vi "Teleop.vi"(10 "Match Info":T1={"Autonomous Elapsed Seconds"=0.0, "TeleOp Elapsed Seconds"=0.0, "Disabled Elapsed Seconds"=0.0, "Visited Autonomous"=FALSE, "Visited TeleOp"=FALSE, "Visited Disabled"=FALSE, "Autonomous Settings"={"Autonomous Style"=enum."Independent", "VI Refnum"=refnum}}, 11 "Call Context":T2=enum."Stop") -> ()   [LabVIEW 2015]
doc: "This VI is called for each TeleOp packet received from the DS where the robot is not disabled. It is often used to read from the joysticks and update I/O or to update setpoints for timed control loops. It should complete and return within 20 milliseconds or it may miss DS packets."
uses:
  <vilib>/Rock Robotics/WPI/DriverStation/WPI_DriverStationDerivedRobotMode.ctl
  <vilib>/Rock Robotics/WPI/DriverStation/WPI_DriverStationMatch Info.ctl
  Typedef/XBox Buttons.ctl
  Typedef/XBox Axis.ctl
  <vilib>/Rock Robotics/WPI/Utilities/WPI_GetSetVariantRefNum.vi
  <vilib>/Rock Robotics/Network Tables/NT Write Boolean Array.vi
  <vilib>/Rock Robotics/Network Tables/NT Write Numeric Array.vi
  Robot Global Data.vi
  <vilib>/Rock Robotics/WPI/RobotDrive/WPI_RobotDriveArcadeDrive_Standard(NoSaturation).vi
  <vilib>/Rock Robotics/Network Tables/NT Write Number.vi
  ArmController/ArmController.lvlib
  <vilib>/Rock Robotics/WPI/Solenoid/WPI_SolenoidSetEnum.vi
  <vilib>/Rock Robotics/WPI/Solenoid/WPI_SolenoidValue.ctl
panel:
  in  "Position":dbl caption="Test Servo Position"
  in  "ServoClose":dbl
  in  "Servo Open":dbl
  in  "Allow Hang":bool
  in  "Winch Speed":dbl=1.0 format="%#_13g"
  in  "Match Time":dbl=115.0 format="%#_13g"
  in  "Reset":bool
  out "Shifts":i32
  # "Hanger"
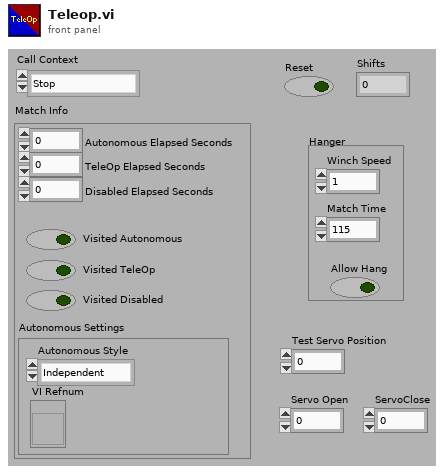
[diagram p1: front panel]
types:
  T1 = typedef "WPI_DriverStationMatch Info.ctl" = cluster{"Autonomous Elapsed Seconds":dbl, "TeleOp Elapsed Seconds":dbl, "Disabled Elapsed Seconds":dbl, "Visited Autonomous":bool, "Visited TeleOp":bool, "Visited Disabled":bool, "Autonomous Settings":cluster{"Autonomous Style":enum16{"Iterative", "Independent"}, "VI Refnum":refnum<vi>}}
  T2 = typedef "WPI_DriverStationDerivedRobotMode.ctl" = enum16{"Init", "Execute", "Stop"}
  T3 = typedef "XBox Buttons.ctl" = enum16{"A", "B", "X", "Y", "Left Bumper", "Right Bumper", "Back", "Start", "Left Joystick", "Right Joystick"}
  T4 = typedef "XBox Axis.ctl" = enum16{"Left X", "Left Y", "Left Trigger", "Right Trigger", "Right X", "Right Y"}
  T5 = typedef "WPI_RobotDriveDevRef.ctl" = cluster{"DevStatus":errorcluster, "Motors[]":T6[], "Square Inputs":bool, "Max Output":dbl}
  T6 = typedef "WPI_MotorControlDeviceRef.ctl" = cluster{"DeviceStatus":errorcluster, "Type":T7, "PWM":cluster{"PWM Channel":T8, "DeadBand":T9}, "CAN":cluster{"Device Number":u8, "Control Mode":T10, "Semaphore":T11, "Max Vout":dbl, "TalonSRX Control Mode":T12}, "Invert":bool}
  T7 = typedef "WPI_MotorControlType.ctl" = enum16{"PWM", "CAN", "CANTalonSRX"}
  T8 = typedef "FPGA_DIOPWMChannel.ctl" = enum8{"PWM 0", "PWM 1", "PWM 2", "PWM 3", "PWM 4", "PWM 5", "PWM 6", "PWM 7", "PWM 8", "PWM 9", "PWM MXP 0", "PWM MXP 1", "PWM MXP 2", "PWM MXP 3", "PWM MXP 4", "PWM MXP 5", "PWM MXP 6", "PWM MXP 7", "PWM MXP 8", "PWM MXP 9", "Invalid"}
  T9 = typedef "WPI_PWMDeadband.ctl" = cluster{"Name":string, "maxPositivePwm":i32, "minPositivePwm":i32, "centerPwm":i32, "maxNegativePwm":i32, "minNegativePwm":i32, "angularRange":u16}
  T10 = typedef "WPI_CANJaguar_ControlMode.ctl" = enum8{"Percent VBus", "Current", "Speed", "Position", "Voltage"}
  T11 = typedef "Semaphore RefNum" = refnum<k1>
  T12 = typedef "WPI_CANTalonSRX_APIControlMode.ctl" = enum8{"Percent VBus", "Speed", "Position", "Slave", "Unchanged / Invalid", "Voltage Compensation", "Current", "Motion Profile"}
  T13 = typedef "WPI_JoystickDevRef.ctl" = cluster{"Device":T14}
  T14 = typedef "WPI_JoystickDeviceEnum.ctl" = enum16{"USB 0", "USB 1", "USB 2", "USB 3", "USB 4", "USB 5"}
  T15 = typedef "WPI_SolenoidValue.ctl" = enum16{"Off", "On", "Forward", "Reverse"}
  T16 = typedef "ArmController.lvlib/ArmRef.ctl" = cluster{"Pot":T17, "ArmMotor":T6, "Queue":refnum<queue>, "Setpoint":dbl, "Manual":bool, "output range":cluster{"output high":dbl, "output low":dbl}, "PID gains":cluster{"proportional gain (Kc)":dbl, "integral time (Ti, min)":dbl, "derivative time (Td, min)":dbl}}
  T17 = typedef "WPI_PotentiometerDevRef.ctl" = cluster{"DevStatus":errorcluster, "Analog Channel":T18, "Invert Output":bool}
  T18 = typedef "FPGA_AIChannel.ctl" = enum8{"AI 0", "AI 1", "AI 2", "AI 3", "AI MXP 0", "AI MXP 1", "AI MXP 2", "AI MXP 3", "Invalid"}
  T19 = typedef "WPI_ServoDeviceRef.ctl" = cluster{"DeviceStatus":errorcluster, "PWM Channel":T8, "DeadBand":T9}
  T20 = cluster{"Down":dbl, "Pickup":dbl, "Shoot":dbl, "Turtle":dbl, "Intake Block":dbl, "Intake Transfer":dbl, "Cheval De Fris":dbl, "Hang":dbl}
  T21 = cluster{"Down":dbl, "Pickup":dbl, "Shoot":dbl, "Turtle":dbl, "Intake Transfer":dbl, "Hang":dbl}
  T22 = typedef "WPI_SolenoidDevRef.ctl" = cluster{"DevStatus":errorcluster, "Pneumatics Control Module":u8, "Forward Solenoid Channel":T23, "Reverse Solenoid Channel":T23}
  T23 = typedef "WPI_SolenoidChannel.ctl" = enum8{"Solenoid 0", "Solenoid 1", "Solenoid 2", "Solenoid 3", "Solenoid 4", "Solenoid 5", "Solenoid 6", "Solenoid 7", "Invalid"}
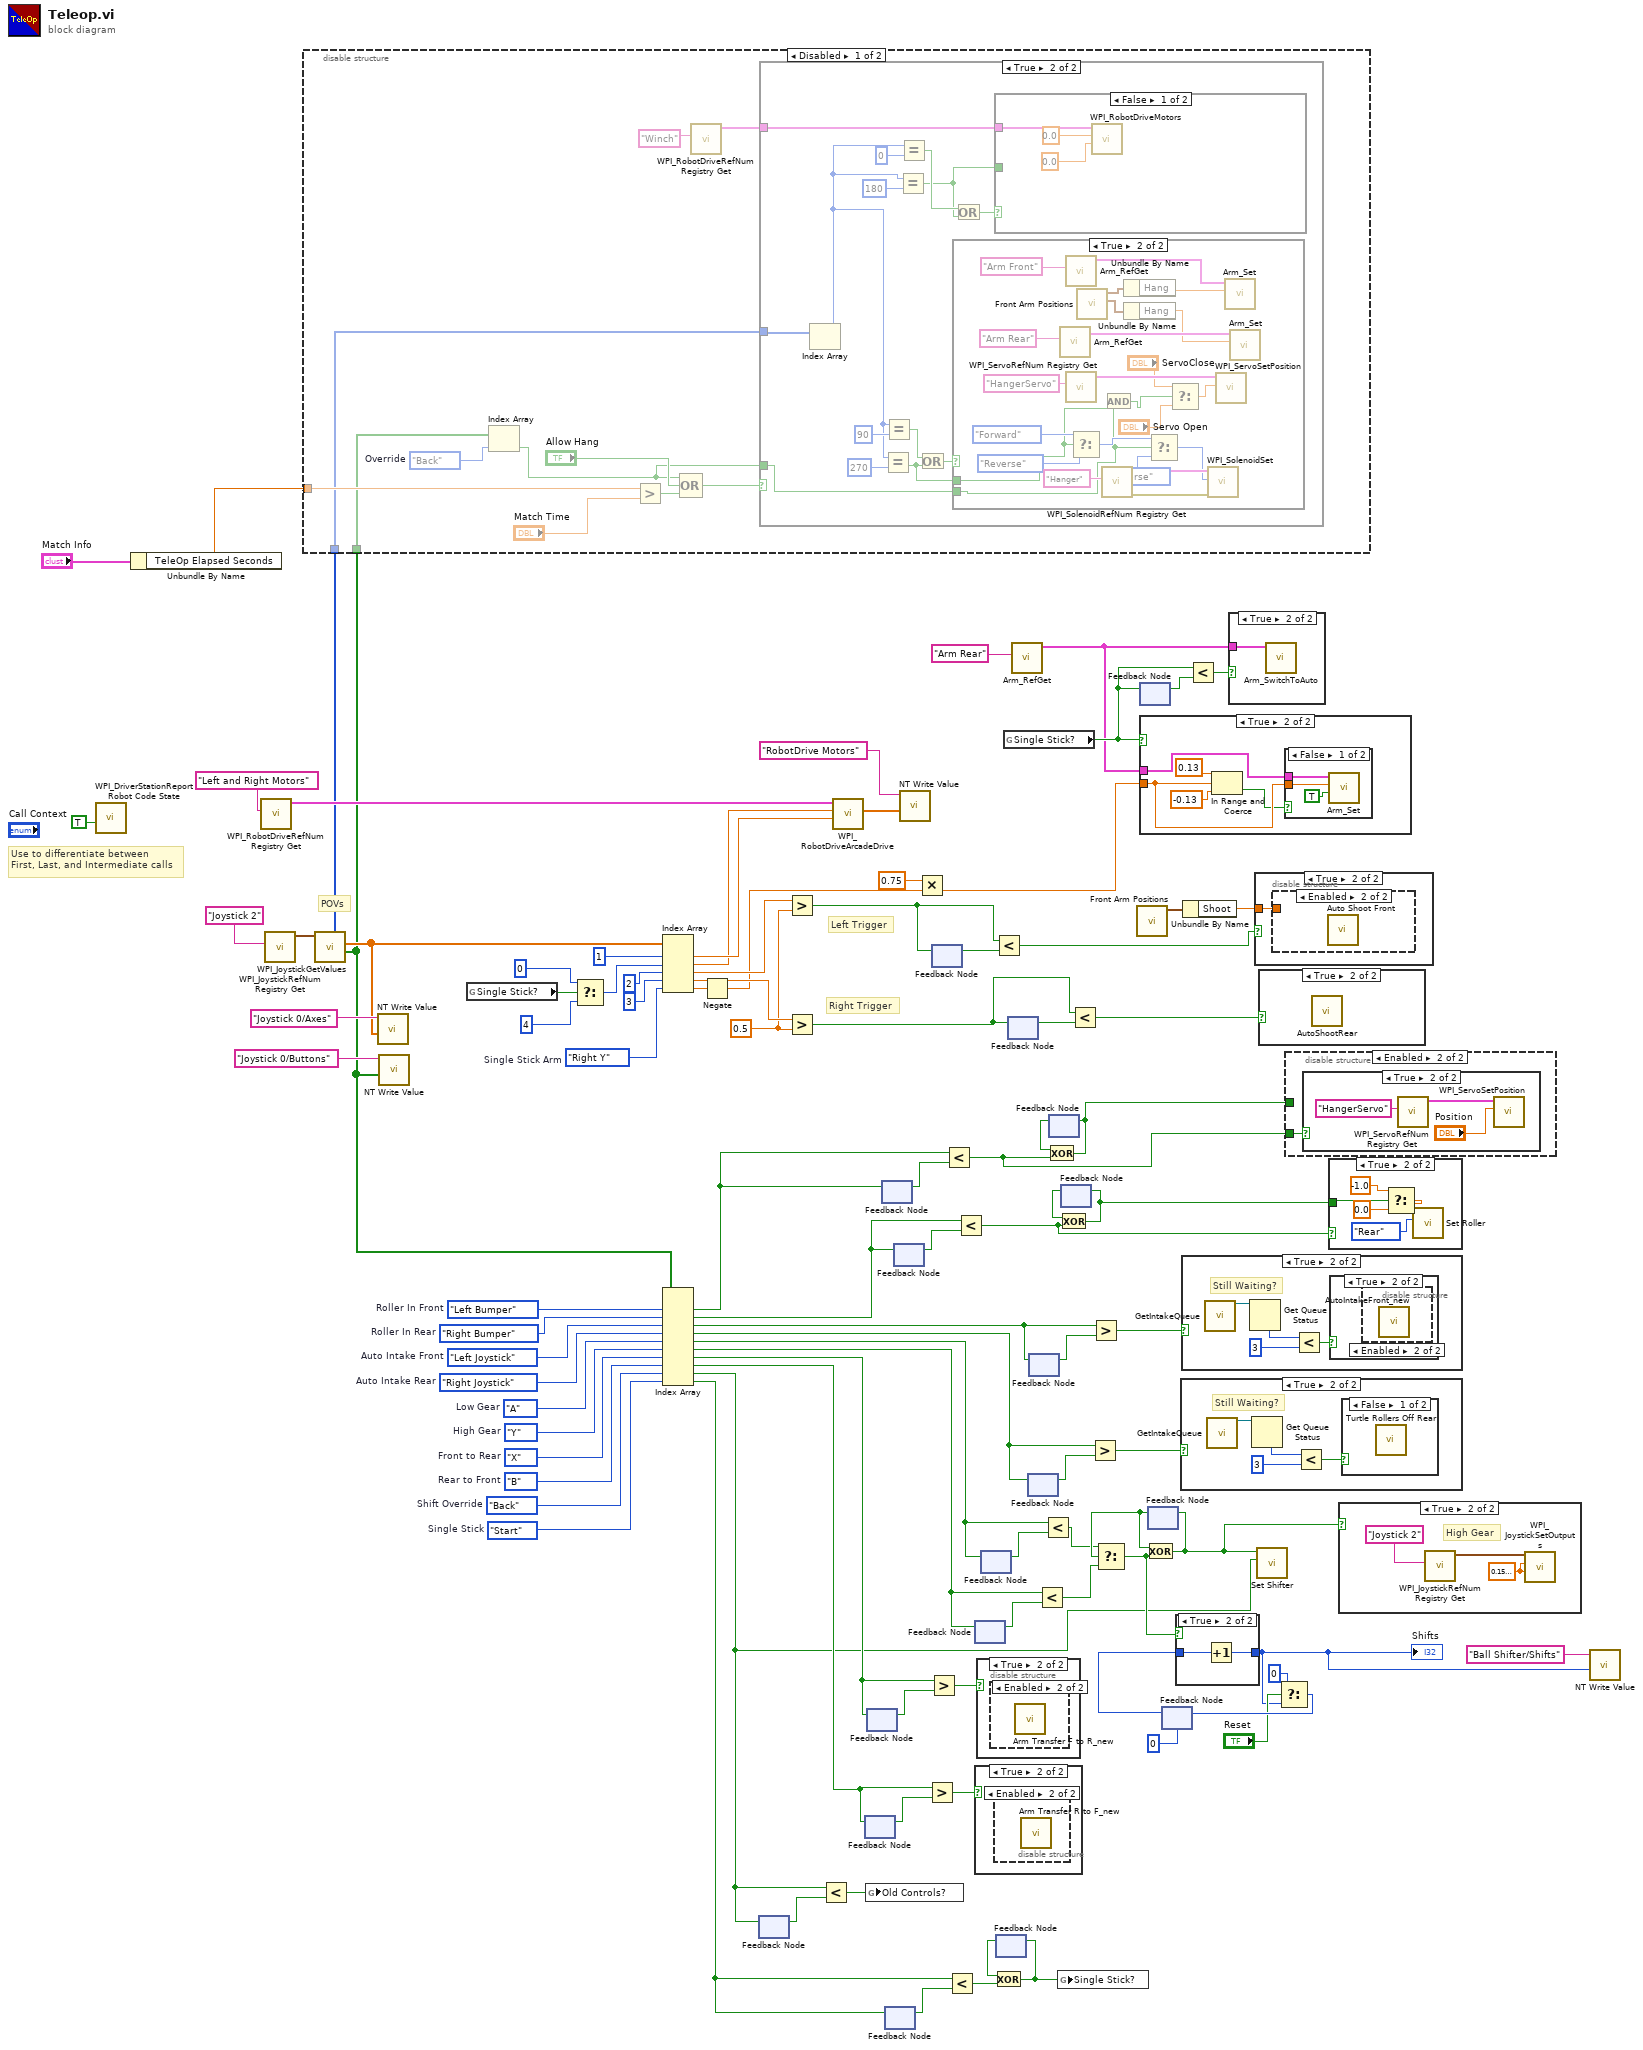
[diagram p0: block diagram]
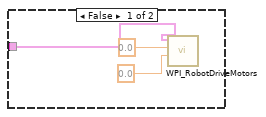
[diagram p2: hidden frame]
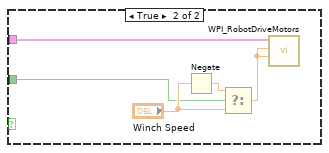
[diagram p4: hidden frame]
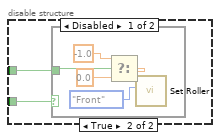
[diagram p6: hidden frame]
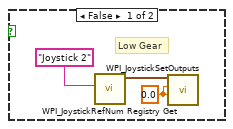
[diagram p9: hidden frame]
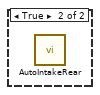
[diagram p11: hidden frame]
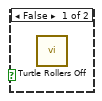
[diagram p13: hidden frame]
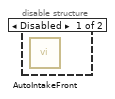
[diagram p14: hidden frame]
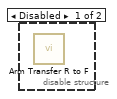
[diagram p16: hidden frame]
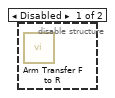
[diagram p20: hidden frame]
diagram:
  w44 = XBox_Buttons."Left Bumper"  # Roller In Front
  w43 = XBox_Buttons."Right Bumper"  # Roller In Rear
  w50 = XBox_Axis."Right Y"  # Single Stick Arm
  w51 = XBox_Buttons."Left Joystick"  # Auto Intake Front
  w52 = XBox_Buttons."Right Joystick"  # Auto Intake Rear
  w53 = XBox_Buttons."A"  # Low Gear
  w54 = XBox_Buttons."Y"  # High Gear
  w55 = XBox_Buttons."X"  # Front to Rear
  w56 = XBox_Buttons."B"  # Rear to Front
  w57 = XBox_Buttons."Back"  # Shift Override
  w58 = XBox_Buttons."Start"  # Single Stick
  w79 = 0.5 ("x")
  # "POVs"
  # "Right Trigger"
  # "Left Trigger"
  # "Use to differentiate between\nFirst, Last, and Intermediate calls"
  n1 = call <vilib>:"WPI_DriverStationReport Robot Code State.vi"("TeleOp"=TRUE ("Autonomous")) -> ()  [unwired: 10 in, 1 out]
  n2 = Unbundle By Name("Match Info") -> ("TeleOp Elapsed Seconds"=w3:dbl)
  n3 = call <vilib>:"WPI_RobotDriveRefNum Registry Get.vi"("refnum name"="Left and Right Motors") -> ("RobotDriveDevRef"=w99:T5)  [unwired: 1 in, 9 out]
  n4 = call <vilib>:"WPI_JoystickRefNum Registry Get.vi"("refnum name"="Joystick 2") -> ("JoystickDevRef"=w6:T13)  [unwired: 1 in, 9 out]
  n5 = call <vilib>:"WPI_JoystickGetValues.vi"("JoystickDevRef"=w6) -> ("Buttons"=w2:bool[], "Axes"=w82:dbl[], "POVs"=w1:i16[])  [unwired: 6 in, 2 out]
  n6 = disable-structure shown="Disabled" {
    disable-tunnel: w3 -> [w111 _]
    disable-tunnel: w2 -> [w105 _]
    disable-tunnel: w1 -> [w104 _]
    frame Disabled {
      w106 = XBox_Buttons."Back"  # Override
      n7 = Index Array(array=w105, index=w106) -> (element=w103:bool)
      n8 = Greater?(x=w111, y="Match Time") -> (0:w108:bool)
      n9 = Compound Arithmetic op=OR(w103, "Allow Hang", w108) -> (w109:bool)
      n10 = call <vilib>:"WPI_RobotDriveRefNum Registry Get.vi"("refnum name"="Winch") -> ("RobotDriveDevRef"=w101:T5)  [unwired: 1 in, 9 out]
      n11 = case shown="True" w109 {
        tunnel: w104 -> [_ w126]
        tunnel: w103 -> [_ w116]
        tunnel: w101 -> [w112 w115]
        frame False {
          n12 = call <vilib>:"WPI_RobotDriveMotors.vi"("RightSpeed"=0.0, "LeftSpeed"=0.0, "RobotDriveDevRef"=w112) -> ()  [unwired: 6 in, 3 out]
        }
        frame True {
          n13 = Index Array(array=w126) -> (element=w121:i16)  [unwired: 1 in]
          n14 = Equal?(x=w121, y=i16 270) -> (x = y?=w117:bool)
          n15 = Equal?(x=w121, y=i16 90) -> (x = y?=w120:bool)
          n16 = Equal?(x=w121, y=i16 180) -> (x = y?=w118:bool)
          n17 = Equal?(x=w121, y=i16 0) -> (x = y?=w119:bool)
          n18 = Or(x=w120, y=w117) -> (x .or. y?=w127:bool)
          n19 = case shown="True" w127 {
            tunnel: w117 -> [_ w132]
            tunnel: w116 -> [_ w133]
            frame False {
            }
            frame True {
              n20 = call "Arm_RefGet.vi"("refnum name"="Arm Rear") -> ("ArmRef"=w144:T16)  [unwired: 9 in, 1 out]
              n21 = call "Arm_RefGet.vi"("refnum name"="Arm Front") -> ("ArmRef"=w145:T16)  [unwired: 9 in, 1 out]
              n22 = call <vilib>:"WPI_ServoRefNum Registry Get.vi"("refnum name"="HangerServo") -> ("ServoDeviceRef"=w135:T19)  [unwired: 9 in, 1 out]
              n23 = Select(t=WPI_SolenoidValue."Forward" ("Direction"), s=w132, f=WPI_SolenoidValue."Reverse" ("Direction")) -> (s? t:f=w139:T15)
              n24 = call "Front Arm Positions.vi"() -> ("Rear Arm"=w148:T20, "Front Arm"=w149:T21)  [unwired: 10 in]
              n25 = call <vilib>:"WPI_SolenoidRefNum Registry Get.vi"("refnum name"="Hanger") -> ("error out"=w150:errorcluster, "SolenoidDevRef"=w152:T22)  [unwired: 9 in]
              n26 = And(x=w132, y=w133) -> (x .and. y?=w134:bool)
              n27 = Unbundle By Name(w149) -> ("Hang"=w142:dbl)
              n28 = Unbundle By Name(w148) -> ("Hang"=w143:dbl)
              n29 = Select(t=w139, s=w133, f=WPI_SolenoidValue."Reverse" ("Direction")) -> (s? t:f=w137:T15)
              n30 = Select(t="ServoClose", s=w134, f="Servo Open") -> (s? t:f=w131:dbl)
              n31 = call-poly <vilib>:"WPI_SolenoidSet.vi"("error in (no error)"=w150, "Value"=w137, "SolenoidDevRef"=w152) -> ()  [unwired: 7 in, 2 out]
              n32 = call <vilib>:"WPI_ServoSetPosition.vi"("Position"=w131, "ServoDeviceRef"=w135) -> ()  [unwired: 8 in, 2 out]
              n33 = call "Arm_Set.vi"("Value"=w142, "ArmRef in"=w145) -> ()  [unwired: 8 in, 2 out]
              n34 = call "Arm_Set.vi"("Value"=w143, "ArmRef in"=w144) -> ()  [unwired: 8 in, 2 out]
            }
          }
          n35 = Or(x=w119, y=w118) -> (x .or. y?=w128:bool)
          n36 = case shown="False" w128 {
            tunnel: w118 -> [_ w157]
            tunnel: w115 -> [w155 w156]
            frame False {
              n37 = call <vilib>:"WPI_RobotDriveMotors.vi"("RightSpeed"=0.0, "LeftSpeed"=0.0, "RobotDriveDevRef"=w155) -> ()  [unwired: 6 in, 3 out]
            }
            frame True {
              n38 = Negate(x="Winch Speed") -> (-x=w159:dbl)
              n39 = Select(t=w159, s=w157, f="Winch Speed") -> (s? t:f=w160:dbl)
              n40 = call <vilib>:"WPI_RobotDriveMotors.vi"("RightSpeed"=w160, "LeftSpeed"=w160, "RobotDriveDevRef"=w156) -> ()  [unwired: 6 in, 3 out]
            }
          }
        }
      }
    }
    frame Enabled {
    }
  }
  n41 = call-poly <vilib>:"NT Write Value.vi"("Numeric Array"=w82, "Name"="Joystick 0/Axes") -> ()  [unwired: 9 in, 1 out]
  n42 = call-poly <vilib>:"NT Write Value.vi"("Boolean Array"=w2, "Name"="Joystick 0/Buttons") -> ()  [unwired: 9 in, 1 out]
  n43 = global read "Robot Global Data.vi" "Single Stick?"() -> (w62:bool)
  n44 = Select(t=0 ("index"), s=w62, f=4 ("index")) -> (s? t:f=w59:i32)
  n45 = Index Array(array=w82, index #1=1 ("index"), index #2=w59, index #3=2 ("index"), index #4=3 ("index"), index #5=w50) -> (element #1=w97:dbl, element #2=w94:dbl, element #3=w81:dbl, element #4=w80:dbl, element #5=w66:dbl)
  n46 = Index Array(array=w2, index #1=w44, index #2=w43, index #3=w51, index #4=w52, index #5=w53, index #6=w54, index #7=w55, index #8=w56, index #9=w57, index #10=w58) -> (element #1=w29:bool, element #2=w28:bool, element #3=w48:bool, element #4=w45:bool, element #5=w41:bool, element #6=w37:bool, element #7=w20:bool, element #8=w9:bool, element #9=w5:bool, element #10=w73:bool)
  n47 = Negate(x=w66) -> (-x=w12:dbl)
  n48 = feedback #1() -> (w35:bool)  [unwired: 1 in]
  n49 = feedback-in #1(w5) -> ()
  n50 = Greater?(x=w81, y=w79) -> (0:w24:bool)
  n51 = Greater?(x=w80, y=w79) -> (0:w17:bool)
  n52 = Less?(x=w5, y=w35) -> (x < y?=w34:bool)
  n53 = call-poly <vilib>:"WPI_RobotDriveArcadeDrive.vi"("Y axis value"=w97, "X axis value"=w94, "RobotDriveDevRef"=w99) -> ("Motor Values"=w96:dbl[])  [unwired: 6 in, 2 out]
  n54 = feedback #2() -> (w10:bool)  [unwired: 1 in]
  n55 = feedback-in #2(w9) -> ()
  n56 = global write "Robot Global Data.vi" "Old Controls?"(w34) -> ()
  n57 = feedback #3() -> (w22:bool)  [unwired: 1 in]
  n58 = feedback-in #3(w20) -> ()
  n59 = feedback #4() -> (w33:bool)  [unwired: 1 in]
  n60 = feedback-in #4(w29) -> ()
  n61 = feedback #5() -> (w74:bool)  [unwired: 1 in]
  n62 = feedback-in #5(w73) -> ()
  n63 = feedback #6() -> (w30:bool)  [unwired: 1 in]
  n64 = feedback-in #6(w28) -> ()
  n65 = call-poly <vilib>:"NT Write Value.vi"("Numeric Array"=w96, "Name"="RobotDrive Motors") -> ()  [unwired: 9 in, 1 out]
  n66 = Multiply(x=0.75, y=w12) -> (x*y=w8:dbl)
  n67 = Greater?(x=w9, y=w10) -> (0:w11:bool)
  n68 = Greater?(x=w20, y=w22) -> (0:w21:bool)
  n69 = feedback #7() -> (w25:bool)  [unwired: 1 in]
  n70 = feedback-in #7(w24) -> ()
  n71 = Less?(x=w29, y=w33) -> (x < y?=w16:bool)
  n72 = Less?(x=w73, y=w74) -> (x < y?=w76:bool)
  n73 = Less?(x=w28, y=w30) -> (x < y?=w13:bool)
  n74 = feedback #8() -> (w39:bool)  [unwired: 1 in]
  n75 = feedback-in #8(w37) -> ()
  n76 = case shown="True" w11 {
    frame False {
    }
    frame True {
      n77 = disable-structure shown="Enabled" {
        frame Disabled {
          n78 = call "Arm Transfer R to F.vi"() -> ()  [unwired: 12 in]
        }
        frame Enabled {
          n79 = call "Arm Transfer R to F_new.vi"() -> ()  [unwired: 12 in]
        }
      }
    }
  }
  n80 = case shown="True" w21 {
    frame False {
    }
    frame True {
      n81 = disable-structure shown="Enabled" {
        frame Disabled {
          n82 = call "Arm Transfer F to R.vi"() -> ()  [unwired: 12 in]
        }
        frame Enabled {
          n83 = call "Arm Transfer F to R_new.vi"() -> ()  [unwired: 12 in]
        }
      }
    }
  }
  n84 = feedback #9() -> (w93:bool)  [unwired: 1 in]
  n85 = feedback-in #9(w41) -> ()
  n86 = Less?(x=w24, y=w25) -> (x < y?=w23:bool)
  n87 = feedback #10() -> (w75:bool)  [unwired: 1 in]
  n88 = Exclusive Or(1:w76, 2:w75) -> (0:w72:bool)
  n89 = feedback-in #10(w72) -> ()
  n90 = global read "Robot Global Data.vi" "Single Stick?"() -> (w70:bool)
  n91 = feedback #11() -> (w19:bool)  [unwired: 1 in]
  n92 = feedback-in #11(w17) -> ()
  n93 = call "Arm_RefGet.vi"("refnum name"="Arm Rear") -> ("ArmRef"=w67:T16)  [unwired: 9 in, 1 out]
  n94 = feedback #12() -> (w46:bool)  [unwired: 1 in]
  n95 = feedback-in #12(w45) -> ()
  n96 = feedback #13() -> (w87:bool)  [unwired: 1 in]
  n97 = feedback-in #13(w48) -> ()
  n98 = Less?(x=w37, y=w39) -> (x < y?=w38:bool)
  n99 = Less?(x=w41, y=w93) -> (x < y?=w40:bool)
  n100 = feedback #14() -> (w32:bool)  [unwired: 1 in]
  n101 = Exclusive Or(1:w16, 2:w32) -> (0:w15:bool)
  n102 = feedback-in #14(w15) -> ()
  n103 = global write "Robot Global Data.vi" "Single Stick?"(w72) -> ()
  n104 = feedback #15() -> (w31:bool)  [unwired: 1 in]
  n105 = Exclusive Or(1:w13, 2:w31) -> (0:w14:bool)
  n106 = feedback-in #15(w14) -> ()
  n107 = Less?(x=w17, y=w19) -> (x < y?=w18:bool)
  n108 = Greater?(x=w45, y=w46) -> (0:w47:bool)
  n109 = Greater?(x=w48, y=w87) -> (0:w49:bool)
  n110 = call "Front Arm Positions.vi"() -> ("Front Arm"=w27:T21)  [unwired: 10 in, 1 out]
  n111 = feedback #16() -> (w71:bool)  [unwired: 1 in]
  n112 = feedback-in #16(w70) -> ()
  n113 = case shown="True" w70 {
    tunnel: w67 -> [_ w163]
    tunnel: w8 -> [_ w162]
    frame False {
    }
    frame True {
      n114 = In Range and Coerce(upper limit=0.13, x=w162, lower limit=-0.13) -> (In Range?=w161:bool)  [unwired: 1 out]
      n115 = case shown="False" w161 {
        tunnel: w163 -> [w168 w169]
        tunnel: w162 -> [w167 _]
        frame False {
          n116 = call "Arm_Set.vi"("Manual Control"=TRUE, "Value"=w167, "ArmRef in"=w168) -> ()  [unwired: 7 in, 2 out]
        }
        frame True {
          n117 = call "Arm_SwitchToAuto.vi"("ArmRef in"=w169) -> ()  [unwired: 9 in, 2 out]
        }
      }
    }
  }
  n118 = feedback #17() -> (w42:bool)  [unwired: 1 in]
  n119 = Select(t=w40, s=w42, f=w38) -> (s? t:f=w36:bool)
  n120 = Exclusive Or(1:w36, 2:w42) -> (0:w4:bool)
  n121 = feedback-in #17(w4) -> ()
  n122 = feedback #18(0) -> (w91:i32)
  n123 = case shown="True" w36 {
    tunnel: w91 -> [w170 w172]
    tunnel: [w170 w171] -> w78
    frame False {
    }
    frame True {
      n124 = Increment(x=w172) -> (x+1=w171:i32)
    }
  }
  "Shifts" <- w78
  n125 = case shown="True" w47 {
    frame False {
    }
    frame True {
      # "Still Waiting?"
      n126 = call "GetIntakeQueue.vi"() -> ("queue out"=w174:refnum<queue>)  [unwired: 11 in]
      n127 = Get Queue Status(queue=w174) -> (# elements in queue=w175:i32)  [unwired: 2 in, 7 out]
      n128 = Less?(x=w175, y=3) -> (x < y?=w173:bool)
      n129 = case shown="False" w173 {
        frame False {
          n130 = call "Turtle Rollers Off Rear.vi"() -> ()  [unwired: 12 in]
        }
        frame True {
          n131 = call "AutoIntakeRear.vi"() -> ()  [unwired: 12 in]
        }
      }
    }
  }
  n132 = case shown="True" w49 {
    frame False {
    }
    frame True {
      # "Still Waiting?"
      n133 = call "GetIntakeQueue.vi"() -> ("queue out"=w180:refnum<queue>)  [unwired: 11 in]
      n134 = Get Queue Status(queue=w180) -> (# elements in queue=w179:i32)  [unwired: 2 in, 7 out]
      n135 = Less?(x=w179, y=3) -> (x < y?=w177:bool)
      n136 = case shown="True" w177 {
        frame False {
          n137 = call "Turtle Rollers Off.vi"() -> ()  [unwired: 12 in]
        }
        frame True {
          n138 = disable-structure shown="Enabled" {
            frame Disabled {
              n139 = call "AutoIntakeFront.vi"() -> ()  [unwired: 12 in]
            }
            frame Enabled {
              n140 = call "AutoIntakeFront_new.vi"() -> ()  [unwired: 12 in]
            }
          }
        }
      }
    }
  }
  n141 = Unbundle By Name(w27) -> ("Shoot"=w26:dbl)
  n142 = Less?(x=w70, y=w71) -> (x < y?=w69:bool)
  n143 = case shown="True" w69 {
    tunnel: w67 -> [_ w181]
    frame False {
    }
    frame True {
      n144 = call "Arm_SwitchToAuto.vi"("ArmRef in"=w181) -> ()  [unwired: 9 in, 2 out]
    }
  }
  n145 = case shown="True" w23 {
    tunnel: w26 -> [_ w182]
    frame False {
    }
    frame True {
      n146 = disable-structure shown="Enabled" {
        disable-tunnel: w182 -> [w184 _]
        frame Disabled {
          n147 = call "Set Arm.vi"("Intake"=enum16{"Front", "Rear"}."Front", "Position"=w184) -> ()  [unwired: 10 in]
        }
        frame Enabled {
          n148 = call "Auto Shoot Front.vi"() -> ()  [unwired: 12 in]
        }
      }
    }
  }
  n149 = call "Set Shifter.vi"("Override?"=w5, "Gear (F = Low Gear)"=w4) -> ()  [unwired: 9 in, 1 out]
  n150 = case shown="True" w18 {
    frame False {
    }
    frame True {
      n151 = call "AutoShootRear.vi"() -> ()  [unwired: 12 in]
    }
  }
  n152 = Select(t=0, s="Reset", f=w78) -> (s? t:f=w89:i32)
  n153 = feedback-in #18(w89) -> ()
  n154 = disable-structure shown="Enabled" {
    disable-tunnel: w16 -> [w186 w192]
    disable-tunnel: w15 -> [w185 _]
    frame Disabled {
      n155 = case shown="True" w186 {
        tunnel: w185 -> [_ w190]
        frame False {
        }
        frame True {
          n156 = Select(t=-1.0 ("Speed"), s=w190, f=0.0) -> (s? t:f=w188:dbl)
          n157 = call "Set Roller.vi"("Intake"=enum16{"Front", "Rear"}."Front", "Speed"=w188) -> ()  [unwired: 10 in]
        }
      }
    }
    frame Enabled {
      n158 = case shown="True" w192 {
        frame False {
        }
        frame True {
          n159 = call <vilib>:"WPI_ServoRefNum Registry Get.vi"("refnum name"="HangerServo") -> ("ServoDeviceRef"=w194:T19)  [unwired: 9 in, 1 out]
          n160 = call <vilib>:"WPI_ServoSetPosition.vi"("Position"="Position", "ServoDeviceRef"=w194) -> ()  [unwired: 8 in, 2 out]
        }
      }
    }
  }
  n161 = case shown="True" w13 {
    tunnel: w14 -> [_ w199]
    frame False {
    }
    frame True {
      n162 = Select(t=-1.0 ("Speed"), s=w199, f=0.0) -> (s? t:f=w197:dbl)
      n163 = call "Set Roller.vi"("Intake"=enum16{"Front", "Rear"}."Rear", "Speed"=w197) -> ()  [unwired: 10 in]
    }
  }
  n164 = case shown="True" w4 {
    frame False {
      w203 = sgl 0.0 ("Right Rumble")
      # "Low Gear"
      n165 = call <vilib>:"WPI_JoystickRefNum Registry Get.vi"("refnum name"="Joystick 2") -> ("JoystickDevRef"=w201:T13)  [unwired: 1 in, 9 out]
      n166 = call <vilib>:"WPI_JoystickSetOutputs.vi"("Right Rumble"=w203, "Left Rumble"=w203, "JoystickDevRef"=w201) -> ()  [unwired: 7 in, 2 out]
    }
    frame True {
      w206 = sgl 0.15 ("Right Rumble")
      # "High Gear"
      n167 = call <vilib>:"WPI_JoystickRefNum Registry Get.vi"("refnum name"="Joystick 2") -> ("JoystickDevRef"=w204:T13)  [unwired: 1 in, 9 out]
      n168 = call <vilib>:"WPI_JoystickSetOutputs.vi"("Right Rumble"=w206, "Left Rumble"=w206, "JoystickDevRef"=w204) -> ()  [unwired: 7 in, 2 out]
    }
  }
  n169 = call-poly <vilib>:"NT Write Value.vi"("Numeric"=w78, "Name"="Ball Shifter/Shifts") -> ()  [unwired: 9 in, 1 out]
